vi "DAQ_TTR Meas Initialize.vi"(0 "Physical Channels":tag, 7 "Global Channels":refnum<k21>, 11 "error in":errorcluster) -> (4 "DAQmx Task Out":refnum<k21>, 15 "error out":errorcluster)   [LabVIEW 2021, in "DAQ_Temperature Thermistor Measurement.lvlib"]
doc: "Initialize analog input channels and obtains a Temperature Thermistor DAQmx task\n\nProvide either Physical channel or Global Channel\nIf both physical and Global channels are provided, Global Channels will take precedence"
uses:
  DAQ_Temperature Thermistor Measurement.lvlib
  <vilib>/DAQmx/create/channels.llb/DAQmx Create Channel (AI-Temperature-Thermistor-Vex).vi
panel:
  # "Inputs"
  # "Outputs"
  # "Overview:\nThis VI initializes an AI Module and provides the Temperature Thermistor DAQmx Task Out\n\nHardware Requirements: A compatible PXI, PCIe, USB, cDAQ or Testscale device\n\nSoftware Requirements: NI DAQmx 2022 Q4 or later\n\nInstructions:\n1. Enter physical channel in which Temperature Thermistor Measurement has to be done in Physical Channels control. (Or) Enter Global channels to use it instead of initiating a new task. User must configure only one input. If both are provided, Global Channels will take precedence.\n2. Get the Temperature Thermistor Measurement task from DAQmx Task Out\n\nNote:\n1. The entered Global channel must belong to Vex Thermistor Typed Analog Input.\n2. User can use the DAQmx Task on other modules to configure and initiate Temperature Thermistor Measurements."
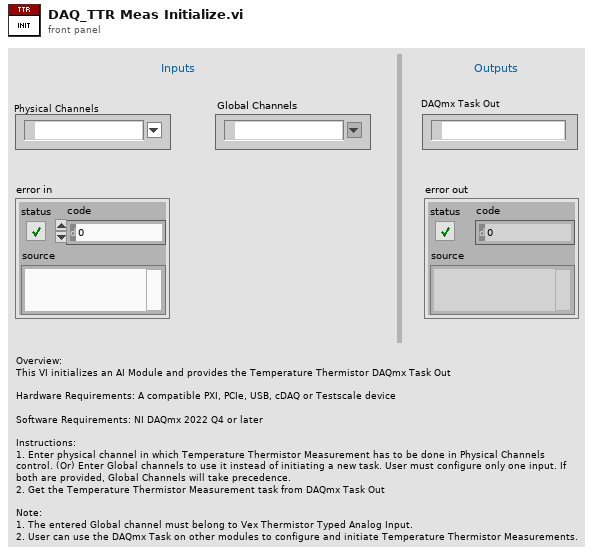
[diagram p1: front panel]
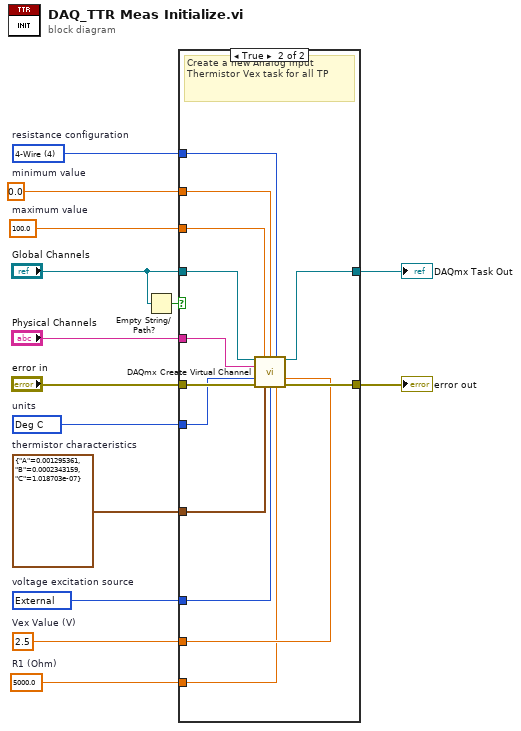
[diagram p0: block diagram]
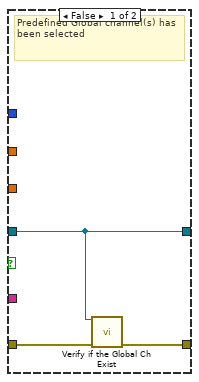
[diagram p2: hidden frame]
diagram:
  w2 = 5000.0  # R1 (Ohm)
  w3 = 10167 items=["Internal"=10200, "External"=10167, "None"=10230]  # voltage excitation source
  w4 = cluster{"A":dbl, "B":dbl, "C":dbl} {"A"=0.001295361, "B"=0.0002343159, "C"=1.018703e-07}  # thermistor characteristics
  w5 = 2.5  # Vex Value (V)
  w6 = 4 items=["2-Wire"=2, "3-Wire"=3, "4-Wire"=4]  # resistance configuration
  w7 = 0.0  # minimum value
  w8 = 100.0  # maximum value
  w9 = 10143 items=["Deg C"=10143, "Deg F"=10144, "Kelvins"=10325, "Deg R"=10145, "From Custom Scale"=10065]  # units
  n1 = Empty String/Path?(string/path="Global Channels") -> (empty?=w11:bool)
  n2 = case shown="True" w11 {
    tunnel: "Physical Channels" -> [_ w27]
    tunnel: "Global Channels" -> [w15 w30]
    tunnel: [w15 w29] -> w1
    tunnel: "error in" -> [w17 w28]
    tunnel: [w16 w26] -> w14
    tunnel: w9 -> [_ w25]
    tunnel: w8 -> [_ w24]
    tunnel: w7 -> [_ w23]
    tunnel: w6 -> [_ w22]
    tunnel: w5 -> [_ w21]
    tunnel: w4 -> [_ w20]
    tunnel: w3 -> [_ w19]
    tunnel: w2 -> [_ w18]
    frame False {
      # "Predefined Global channel(s) has been selected"
      n3 = call "Verify if the Global Ch Exist.vi"("Global Channels"=w15, "error in (no error)"=w17) -> ("error out"=w16:errorcluster)  [unwired: 13 in]
    }
    frame True {
      # "Create a new Analog input Thermistor Vex task for all TP"
      n4 = call-poly <vilib>:"DAQmx Create Virtual Channel.vi"("task in"=w30, "maximum value"=w24, "minimum value"=w23, "resistance configuration"=w22, "physical channels"=w27, "units"=w25, "voltage excitation value"=w21, "error in"=w28, "thermistor characteristics"=w20, "voltage excitation source"=w19, "r1"=w18) -> ("task out"=w29:refnum<k21>, "error out"=w26:errorcluster)  [unwired: 3 in]
    }
  }
  "DAQmx Task Out" <- w1
  "error out" <- w14
